vi "filenoerror.vi"(0 "记录文件路径":path) -> ()   [LabVIEW 2018]
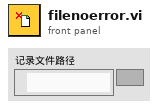
[diagram p1: front panel]
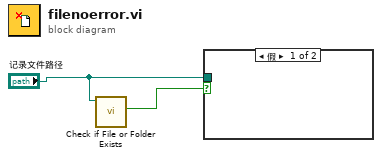
[diagram p0: block diagram]
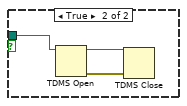
[diagram p2: hidden frame]
diagram:
  n1 = call <vilib>:"Check if File or Folder Exists.vi"("path"="记录文件路径") -> ("file or folder exists?"=w1:bool)  [unwired: 8 in, 2 out]
  n2 = case shown="假" w1 {
    tunnel: "记录文件路径" -> [_ w5]
    frame False {
    }
    frame True {
      n3 = TDMS Open(11:w5) -> (0:w3:errorcluster, 3:w4:refnum<k34>)  [unwired: 6 in]
      n4 = TDMS Close(8:w3, 11:w4) -> ()  [unwired: 2 out]
    }
  }
